vi "Add zero.vi"(8 "error in (no error)":errorcluster, 11 "String in":string) -> (0 "error out":errorcluster, 3 "String out":string)   [LabVIEW 2015, in "LSR Transmission.lvlib"]
uses:
  LSR Transmission.lvlib
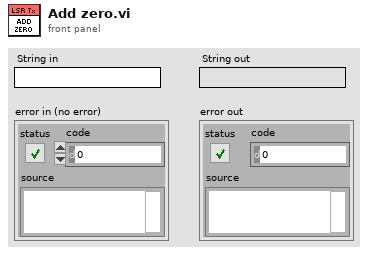
[diagram p1: front panel]
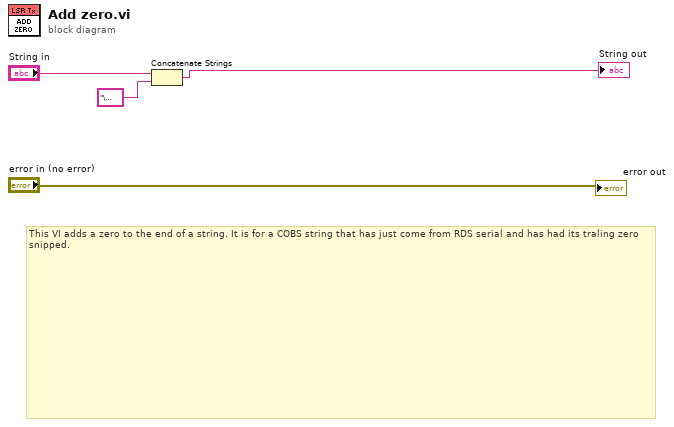
[diagram p0: block diagram]
diagram:
  # "This VI adds a zero to the end of a string. It is for a COBS string that has just come from RDS serial and has had its traling zero snipped."
  n1 = Concatenate Strings("String in", "\u0000" ("string")) -> (→"String out":string)
  "error out" <- "error in (no error)"
